vi "Thruster control commnd algorithm.vi"(3 "RPM Measured":dbl=1.0, 4 "RPM Set":dbl=1.0) -> (0 "Estimated Force":dbl=1.492471782203008 format="%#.3f", 1 "Control Voltage":dbl=1.492471782203008 format="%#.3f")   [LabVIEW 2021]
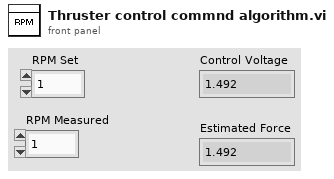
[diagram p1: front panel]
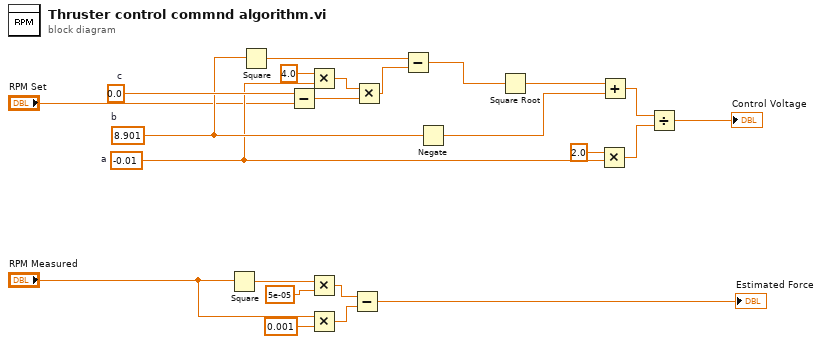
[diagram p0: block diagram]
diagram:
  w23 = 0.0  # c
  w9 = -0.01  # a
  w22 = 8.901  # b
  n1 = Square(x="RPM Measured") -> (x^2=w3:dbl)
  n2 = Square(x=w22) -> (x^2=w21:dbl)
  n3 = Subtract(x=w23, y="RPM Set") -> (x-y=w12:dbl)
  n4 = Multiply(x=4.0, y=w9) -> (x*y=w18:dbl)
  n5 = Multiply(x=w3, y=5e-05) -> (x*y=w7:dbl)
  n6 = Multiply(x="RPM Measured", y=0.001) -> (x*y=w6:dbl)
  n7 = Subtract(x=w7, y=w6) -> (x-y=→"Estimated Force":dbl)
  n8 = Multiply(x=w18, y=w12) -> (x*y=w20:dbl)
  n9 = Subtract(x=w21, y=w20) -> (x-y=w17:dbl)
  n10 = Negate(x=w22) -> (-x=w15:dbl)
  n11 = Square Root(x=w17) -> (sqrt(x)=w16:dbl)
  n12 = Multiply(x=2.0, y=w9) -> (x*y=w13:dbl)
  n13 = Add(x=w16, y=w15) -> (x+y=w14:dbl)
  n14 = Divide(x=w14, y=w13) -> (x/y=→"Control Voltage":dbl)
